vi "Serial Decoder Read Only.vi"(1 "milliseconds to wait":u32=500, 2 "Com Parms":T1={"VISA resource name"="COM6", "baud rate"=38400, "data bits"=8, "parity"=0, "stop bits"=10, "flow control"=0} {"flow control" items=["None"=0, "XON/XOFF"=1, "RTS/CTS"=2, "DTR/DSR"=4]; "stop bits" items=["1.0"=10, "1.5"=15, "2.0"=20]; "parity" items=["None", "Odd", "Even", "Mark", "Space"]; "data bits" min=5 max=8 step=1}, 3 "error in":errorcluster={"status"=FALSE, "code"=-1073807343, "source"=""}) -> (5 "Data Read":T2={"Date"="03/29/13", "Time"="14:47:22", "CO2- ppm"=753, "Last Ctrl Word"=5276928, "O2-1 ppm"=209104, "O2-2 ppm"=209104, "Temp MB"=20.41, "Temp Sensor Modulr"=21.85, "Press mB"=835.52} {"Last Ctrl Word" format="%.0x"}, 7 "error out":errorcluster={"status"=FALSE, "code"=-1073807343, "source"=""})   [LabVIEW 2012]
panel:
  out "read buffer":string="03/29/13,14:47:22,753, 00508500, 209104, 209104, 20.41, 21.85, 835.52\r\n"
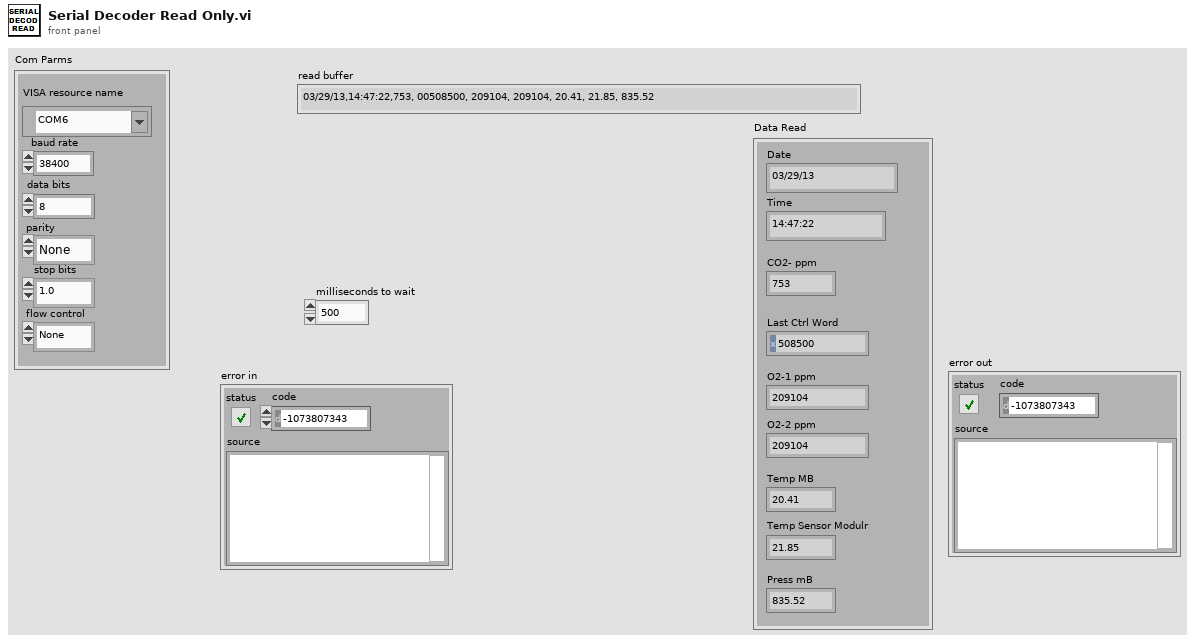
[diagram p1: front panel]
types:
  T1 = cluster{"VISA resource name":refnum<visa-resource-name>, "baud rate":u32, "data bits":u16, "parity":u16, "stop bits":u16, "flow control":u16}
  T2 = cluster{"Date":string, "Time":string, "CO2- ppm":u32, "Last Ctrl Word":u32, "O2-1 ppm":u32, "O2-2 ppm":u32, "Temp MB":sgl, "Temp Sensor Modulr":sgl, "Press mB":sgl}
  T3 = cluster{"default value 1":string, "default value 1":string, "default value 5":u32, "default value 5":u32, "default value 5":u32, "default value 5":u32, "default value 7":sgl, "default value 7":sgl, "default value 7":sgl}
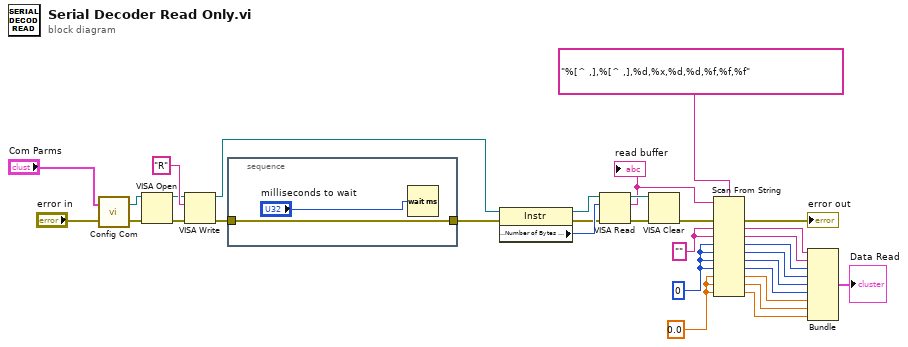
[diagram p0: block diagram]
diagram:
  w9 = sgl 0.0 ("default value 7")
  w22 = "" ("default value 1")
  w4 = u32 0 ("default value 5")
  n1 = call "Config Com.vi"("error in"="error in", "Com Parms"="Com Parms") -> ("error out"=w7:errorcluster, "VISA resource name out"=w8:refnum<visa-resource-name>)
  n2 = VISA Open(error in (no error)=w7, VISA resource name=w8) -> (VISA resource name=w2:refnum<visa-resource-name>, error out=w1:errorcluster)  [unwired: 3 in]
  n3 = VISA Write(VISA resource name=w2, write buffer="R" ("string"), error in (no error)=w1) -> (VISA resource name out=w20:refnum<visa-resource-name>, error out=w21:errorcluster)  [unwired: 1 out]
  n4 = stacked-sequence {
    tunnel: [w33] -> w23
    tunnel: w21 -> [w33]
    frame #0 {
      n5 = Wait (ms)(milliseconds to wait="milliseconds to wait") -> ()  [unwired: 1 out]
    }
  }
  n6 = property class="Instr"(reference=w20, error in=w23) -> (reference out=w25:refnum<visa-resource-name>, error out=w24:errorcluster, "Serial Settings:Number of Bytes at Serial Port"=w26:u32)
  n7 = VISA Read(VISA resource name=w25, byte count=w26, error in (no error)=w24) -> (VISA resource name out=w31:refnum<visa-resource-name>, read buffer=w30:string, error out=w29:errorcluster)  [unwired: 1 out]
  "read buffer" <- w30
  n8 = VISA Clear(VISA resource name=w31, error in (no error)=w29) -> (error out=w28:errorcluster)  [unwired: 1 out]
  n9 = Scan From String(format string="%[^ ,],%[^ ,],%d,%x,%d,%d,%f,%f,%f" ("String"), input string=w30, error in=w28, default 1=w22, default 2=w22, default 3=w4, default 4=w4, default 5=w4, default 6=w4, default 7=w9, default 8=w9, default 9=w9) -> (error out=→"error out":errorcluster, output 1=w19:string, output 2=w18:string, output 3=w17:u32, output 4=w16:u32, output 5=w15:u32, output 6=w14:u32, output 7=w13:sgl, output 8=w12:sgl, output 9=w11:sgl)  [unwired: 1 in, 2 out]
  n10 = Bundle("default value 1"=w19, "default value 1"=w18, "default value 5"=w17, "default value 5"=w16, "default value 5"=w15, "default value 5"=w14, "default value 7"=w13, "default value 7"=w12, "default value 7"=w11) -> (→"Data Read":T3)  [unwired: 1 in]
